vi "Test FTDI SPI SYS Set.vi"() -> ()   [LabVIEW 2018]
uses:
  PROJEKT/NIKO/Labview/Niko V4/FTDI SPI/Ctl/Sub Addr.ctl
panel:
  in  "nCS":u8 max=4 step=1
  out "Latch Reg":u16
  in  "Addr":T1 items=["Addr-0", "Addr-1", "Addr-2", "Addr-3", "Addr-4", "Addr-5", "Addr-6", "Addr-7"]
  out "error out":errorcluster
  in  "Relays (1-10)":bool[](array[boolean])=[FALSE, FALSE, FALSE, FALSE, FALSE, FALSE, FALSE, FALSE, FALSE, FALSE]
  out "Ini Status":bool
  in  "config":T2={"ClockRate"=50000, "LatencyTimer"=10, "configOptions 24-31"=0, "configOptions 16-23"=0, "configOptions 8-15"=0, "configOptions 0-7"=32, "Pin"=0, "reserved"=0} {"configOptions 24-31" format="%x"; "configOptions 16-23" format="%x"; "configOptions 8-15" format="%x"; "configOptions 0-7" format="%x"}
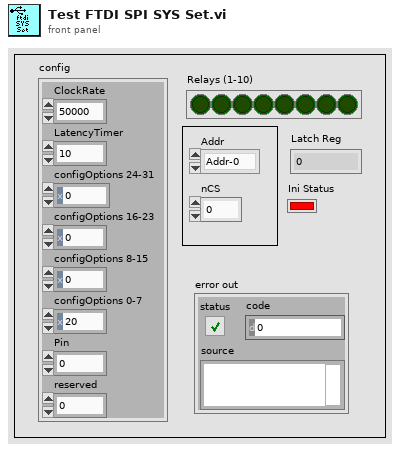
[diagram p1: front panel]
types:
  T1 = typedef "Sub Addr.ctl" = u16
  T2 = cluster{"ClockRate":u32, "LatencyTimer":u8, "configOptions 24-31":i8, "configOptions 16-23":i8, "configOptions 8-15":i8, "configOptions 0-7":u32, "Pin":u32, "reserved":u16}
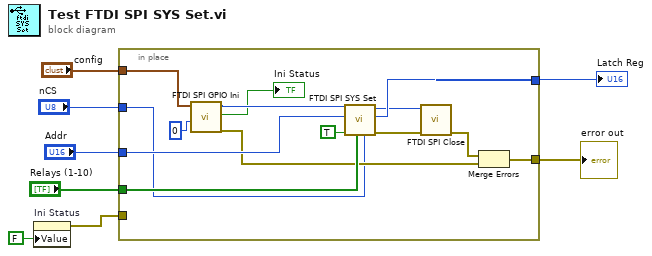
[diagram p0: block diagram]
diagram:
  n1 = property on="Ini Status" class="Bool (strict)"("Value"=FALSE ("Ini Status")) -> (error out=w4:errorcluster)  [unwired: 2 in, 1 out]
  n2 = in-place {
    in-place-border: "config" -> [w10]
    in-place-border: "Addr" -> [w21]
    in-place-border: "Relays (1-10)" -> [w20]
    in-place-border: w4 -> [_]
    in-place-border: [w19] -> w3
    in-place-border: [w11] -> w2
    in-place-border: "nCS" -> [w9]
    n3 = call "FTDI SPI GPIO Ini.vi"("Channel Nmb"=u8 0 ("FTDI Dev Nmb"), "config"=w10) -> ("error out"=w15:errorcluster, "Ini Status"=→"Ini Status":bool, "handle out"=w17:u32)  [unwired: 5 in, 2 out]
    n4 = call "FTDI SPI SYS Set.vi"("nCS"=w9, "Set Out (0-7)"=w20, "Use Extra"=TRUE, "Addr"=w21, "Handler In"=w17) -> ("error out"=w13:errorcluster, "Latch Reg"=w19:u32, "Handler Out"=w14:u32)  [unwired: 4 in]
    n5 = call "FTDI SPI Close.vi"("error in (no error)"=w13, "Handler In"=w14) -> ("error out"=w12:errorcluster)  [unwired: 9 in]
    n6 = Merge Errors(w12, w15) -> (w11:errorcluster)
  }
  "Latch Reg" <- w3
  "error out" <- w2
